vi "Linear Fit Coefficients (LAR).vi"(0 "Y":dbl[](array[numeric]) format="%#.6g", 5 "X":dbl[](array[numeric]) format="%#.6g", 7 "Weight":dbl[](array[numeric]) format="%#.6g", 9 "tol":dbl=0.0001) -> (4 "slope":dbl format="%#.6g", 6 "intercept":dbl format="%#.6g", 15 "error":i32)   [LabVIEW 2017, in "NI_AALPro.lvlib"]
uses:
  NI_AALPro.lvlib
  lvanlys.dll
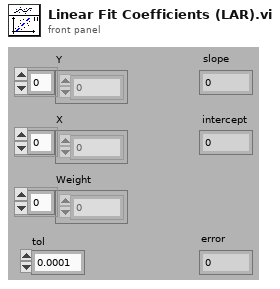
[diagram p1: front panel]
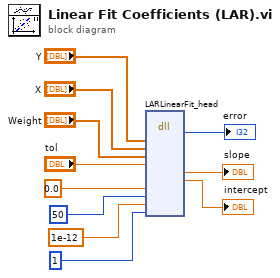
[diagram p0: block diagram]
diagram:
  n1 = dll-call lib="C:/Program Files/National Instruments/LabVIEW 2017/resource/lvanlys.*" fn="LARLinearFit_head"("yH"="Y", "xH"="X", "weight"="Weight", "tol"="tol", "meanErr"=0.0, "maxIter"=50, "absTol"=1e-12, "isCoef"=1) -> (→"error":i32, "slope"=→"slope":dbl, "intercept"=→"intercept":dbl)  [unwired: 13 in, 2 out]
